vi "ADS Create TCV.vi"(4 "iou":dbl, 6 "conf":dbl, 7 "Width":u32, 9 "model_w":i32, 10 "model_h":i32, 11 "Height":u32) -> (0 "error out":errorcluster, 3 "Ref out":u64)   [LabVIEW 2024]
uses:
  TransformCV-LabVIEW/Test/dependencies_dll_release/TCV_Lib.dll
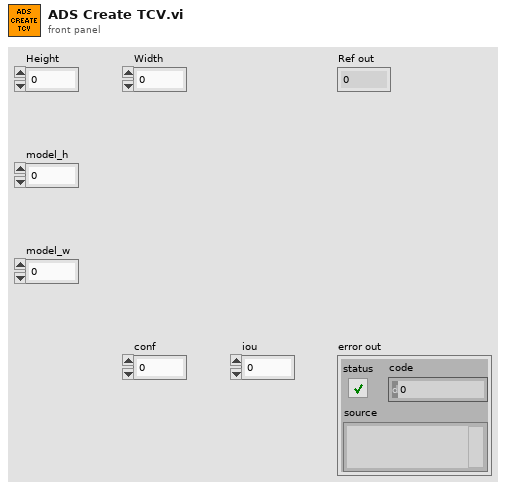
[diagram p1: front panel]
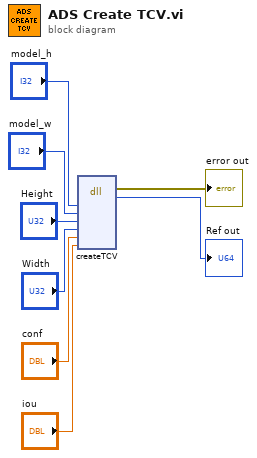
[diagram p0: block diagram]
diagram:
  n1 = dll-call lib="D:/TransformCV-LabVIEW/Test/dependencies_dll_release/TCV_Lib.dll" fn="createTCV"("model_h"="model_h", "model_w"="model_w", "frame_h"="Height", "frame_w"="Width", "conf"="conf", "iou"="iou") -> (error out=→"error out":errorcluster, "return Obj"=→"Ref out":u64)  [unwired: 9 in, 1 out]
